vi "Router - PXImc Open.vi"(8 "error in (no error)":errorcluster, 11 "Router Data In":T1) -> (0 "error out":errorcluster, 3 "Router Data Out":T1)   [LabVIEW 2016, in "PXImc Router.lvlib"]
uses:
  PXImc Router.lvlib
  Controls/Router/Router - Config.ctl
  Controls/Router/Router - Node Block R-W Properties.ctl
  Controls/Router/Router - Block Properties.ctl
  Controls/Router/Router - PXImc Properties.ctl
  Controls/Router/Router - PXImc Card Properties.ctl
  <vilib>/pximc/Initialize Reader Session (U8).vi
  <vilib>/pximc/Initialize Writer Session (U8).vi
  <vilib>/pximc/nipximc.lvlib
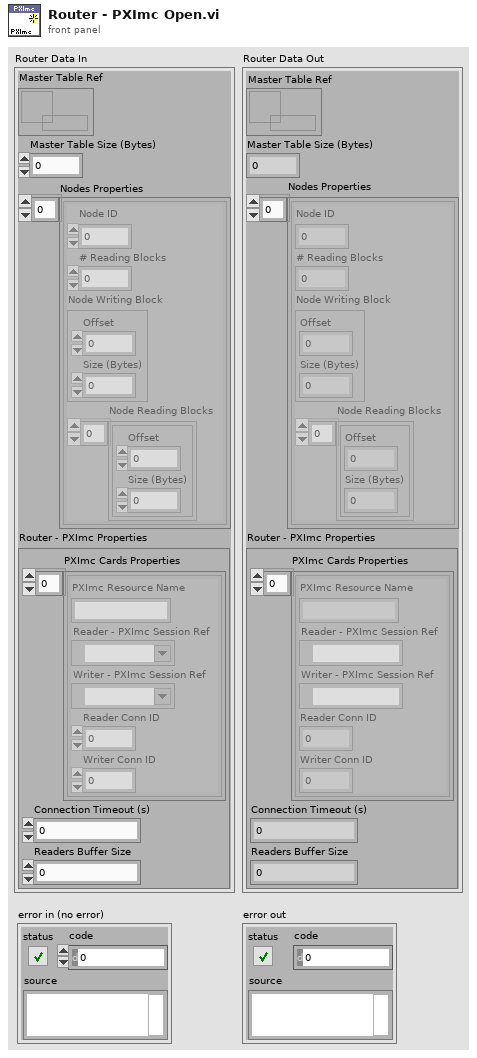
[diagram p1: front panel]
types:
  T1 = typedef "PXImc Router.lvlib/Router - Config.ctl" = cluster{"Master Table Ref":refnum<data-value>, "Master Table Size (Bytes)":u32, "Nodes Properties":T2[], "Router - PXImc Properties":T4}
  T2 = typedef "PXImc Router.lvlib/Router - Node Block R-W Properties.ctl" = cluster{"Node ID":u32, "# Reading Blocks":u32, "Node Writing Block":T3, "Node Reading Blocks":T3[]}
  T3 = typedef "PXImc Router.lvlib/Router - Block Properties.ctl" = cluster{"Offset":u32, "Size (Bytes)":u32}
  T4 = typedef "PXImc Router.lvlib/Router - PXImc Properties.ctl" = cluster{"PXImc Cards Properties":T5[], "Connection Timeout (s)":dbl, "Readers Buffer Size":u64}
  T5 = typedef "PXImc Router.lvlib/Router - PXImc Card Properties.ctl" = cluster{"PXImc Resource Name":string, "Reader - PXImc Session Ref":refnum<k21>, "Writer - PXImc Session Ref":refnum<k21>, "Reader Conn ID":u16, "Writer Conn ID":u16}
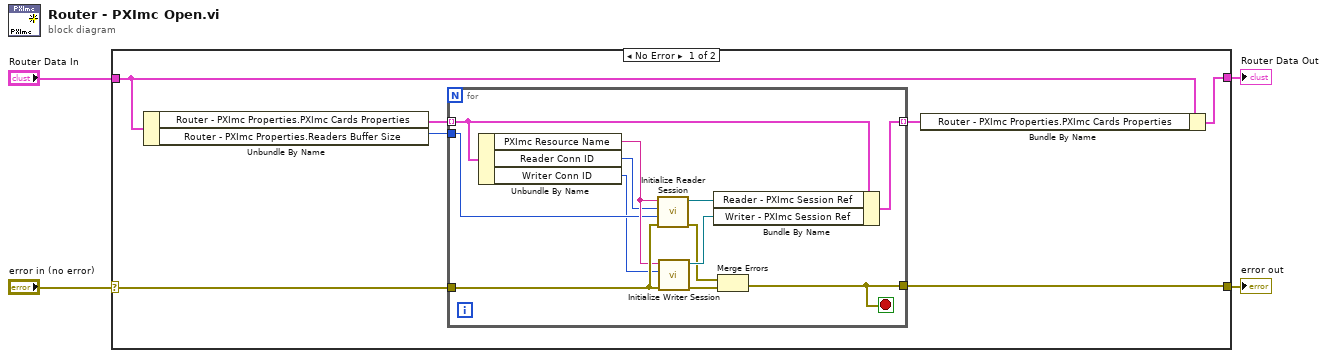
[diagram p0: block diagram]
diagram:
  n1 = case shown="No Error" "error in (no error)" {
    selector: "error in (no error)" -> [w10 w24]
    tunnel: "Router Data In" -> [w9 w25]
    tunnel: [w11 w25] -> w1
    tunnel: [w5 w24] -> w4
    frame No Error {
      n2 = Unbundle By Name(w9) -> ("Router - PXImc Properties.PXImc Cards Properties"=w8:T5[], "Router - PXImc Properties.Readers Buffer Size"=w7:u64)
      n3 = for {
        tunnel: w8 -> [w18] mode=indexing
        tunnel: w7 -> [w20]
        tunnel: [w15] -> w6 mode=indexing
        tunnel: w10 -> [w23]
        tunnel: [w12] -> w5
        stop <- w12 stop-if-true
        n4 = Unbundle By Name(w18) -> ("PXImc Resource Name"=w22:string, "Reader Conn ID"=w21:u16, "Writer Conn ID"=w19:u16)
        n5 = call-poly <vilib>:"Initialize Reader Session.vi"("error in (no error)"=w23, "buffer size"=w20, "writer's connection id (1)"=w21, "interface"=w22) -> ("error out"=w14:errorcluster, "session out"=w17:refnum<k21>)  [unwired: 6 in]
        n6 = call-poly <vilib>:"Initialize Writer Session.vi"("error in (no error)"=w23, "connection id (1)"=w19, "interface"=w22) -> ("error out"=w13:errorcluster, "session out"=w16:refnum<k21>)  [unwired: 7 in]
        n7 = Bundle By Name(cluster=w18, "Reader - PXImc Session Ref"=w17, "Writer - PXImc Session Ref"=w16) -> (w15:T5)
        n8 = Merge Errors(w14, w13) -> (w12:errorcluster)
      }
      n9 = Bundle By Name(cluster=w9, "Router - PXImc Properties.PXImc Cards Properties"=w6) -> (w11:T1)
    }
    frame Error {
    }
  }
  "error out" <- w4
  "Router Data Out" <- w1
